vi "UDP Rx Launch.vi"(5 "max size (548)":i32, 7 "port":u16, 8 "error in (no error)":errorcluster, 11 "Stop Pointer":refnum<class "Pointer.lvclass">) -> (0 "error out":errorcluster, 3 "Count Pointer":refnum<class "Pointer.lvclass">)   [LabVIEW 2019]
uses:
  <vilib>/NI/Memory Manager/Classes/Pointer/Pointer.lvclass
  <vilib>/NI/Memory Manager/Classes/Pointer/Pointer.lvclass/Pointer.ctl
  <vilib>/NI/Memory Manager/Classes/Pointer/Write U32.vi
  <vilib>/NI/Memory Manager/Classes/Pointer/Set Address.vi
  <vilib>/NI/Memory Manager/Classes/Pointer/Set Size.vi
  <vilib>/NI/Memory Manager/Classes/Pointer/Set Internal.vi
  <vilib>/NI/Memory Manager/Classes/Pointer/Write (No Check).vi
  <vilib>/NI/Memory Manager/Classes/Pointer/Write (No Check) U32.vi
  <vilib>/NI/Memory Manager/Classes/Pointer/Check Move.vi
  <vilib>/NI/Memory Manager/Classes/Pointer/Get Address.vi
  <vilib>/NI/Memory Manager/Classes/Pointer/Check Null Pointer.vi
  <vilib>/NI/Memory Manager/Classes/Pointer/Check Count.vi
  <vilib>/NI/Memory Manager/Classes/Pointer/Check Bounds (Power of 2).vi
  <vilib>/NI/Memory Manager/Classes/Pointer/Errors.vi
  <vilib>/NI/Memory Manager/Classes/Pointer/Null Pointer.vi
  <vilib>/NI/Memory Manager/Classes/Pointer/Is Null.vi
  <vilib>/NI/Memory Manager/Classes/Pointer/Get Size.vi
  <vilib>/NI/Memory Manager/Classes/Pointer/Out of Bounds.vi
  <vilib>/NI/Memory Manager/Classes/Pointer/Check Bounds.vi
  <vilib>/NI/Memory Manager/Classes/Pointer/Create Error.vi
  <vilib>/NI/Memory Manager/VIs/Write String to Source.vi
  <vilib>/NI/Memory Manager/Classes/Pointer/Write Pointer Size to Error.vi
  <vilib>/NI/Memory Manager/VIs/Write Numeric to Source.vi
  <vilib>/NI/Memory Manager/VIs/Write Numeric Scalar to Source (Base10 U64).vi
  <vilib>/NI/Memory Manager/Classes/Pointer/Check Bounds (Pointer).vi
  <vilib>/NI/Memory Manager/Classes/Pointer/Check Bounds (Buffer).vi
  <vilib>/NI/Memory Manager/VIs/New Error Cluster.vi
  <vilib>/NI/Memory Manager/VIs/New Error Cluster (512B).vi
  <vilib>/NI/Memory Manager/VIs/Set Error Status.vi
  <vilib>/NI/Memory Manager/VIs/Set Error Code.vi
  <vilib>/NI/Memory Manager/VIs/Set Error Source.vi
  <vilib>/NI/Memory Manager/Constants/Constants.vi
  <vilib>/NI/Memory Manager/Constants/Library Name.vi
  <vilib>/NI/Memory Manager/Classes/Pointer/Pointer Error Info.vi
  <vilib>/NI/Memory Manager/Constants/Pointer Class Name.vi
  <vilib>/NI/Memory Manager/Classes/Pointer/Buffer Underflow.vi
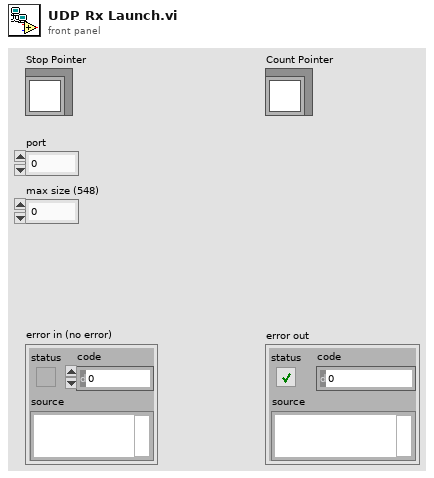
[diagram p1: front panel]
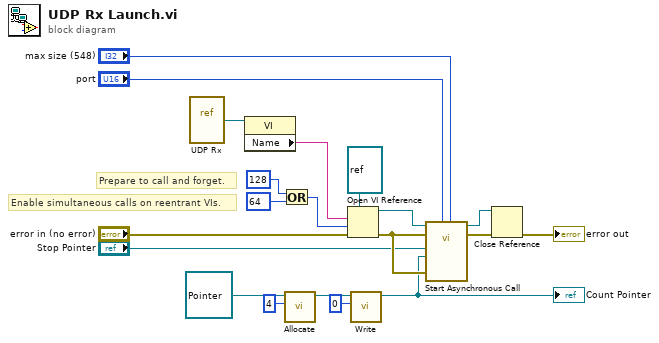
[diagram p0: block diagram]
diagram:
  # "Prepare to call and forget."
  # "Enable simultaneous calls on reentrant VIs."
  n1 = vi-ref "UDP Rx.vi"() -> (w10:refnum<vi>)
  n2 = property class="VI"(reference=w10) -> ("Name"=w11:string)  [unwired: 1 in, 2 out]
  n3 = Or(x=128 ("options"), y=64 ("options")) -> (x .or. y?=w13:i32)
  n4 = call <vilib>:"Allocate.vi"("size"=u64 4, "Pointer type"=refnum<class "Pointer.lvclass"> refnum ("Pointer in")) -> ("Pointer out"=w3:refnum<class "Pointer.lvclass">)  [unwired: 8 in, 1 out]
  n5 = Open VI Reference(type specifier VI Refnum (for type only)=refnum<vi> refnum, vi path=w11, options=w13, error in (no error)="error in (no error)") -> (vi reference=w18:refnum<vi>, error out=w20:errorcluster)  [unwired: 2 in]
  n6 = call-poly <vilib>:"Write.vi"("value"=u32 0, "Pointer in"=w3) -> ("Pointer out"=w2:refnum<class "Pointer.lvclass">)  [unwired: 6 in, 3 out]
  "Count Pointer" <- w2
  n7 = call-by-ref "Start Asynchronous Call"(reference=w18, error in=w20, "max size (548)"="max size (548)", "port"="port", 8:"error in (no error)"=w20, "Count Pointer"=w2, "Stop Pointer"="Stop Pointer") -> (reference out=w16:refnum<vi>, error out=w17:errorcluster)  [unwired: 6 in, 1 out]
  n8 = Close Reference(reference=w16, error in (no error)=w17) -> (error out=→"error out":errorcluster)
